vi "create unique name.vi"(10 "UID":string, 11 "alias":string) -> (3 "unique ring name":string)   [LabVIEW 2013, in "PL Framework Configuration Tool.lvlib" / "Engine Mappings.lvclass"]
uses:
  Engine Mappings.lvclass
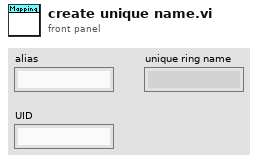
[diagram p1: front panel]
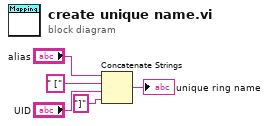
[diagram p0: block diagram]
diagram:
  n1 = Concatenate Strings("alias", " [" ("string"), "UID", "]" ("string")) -> (→"unique ring name":string)
